vi "RotApp_SaveConfig.vi"(11 "configuration file":path) -> ()   [LabVIEW 2012]
uses:
  RotationProgram/Global/RotationGlobal.vi
  <vilib>/Utility/config.llb/Write Key (Double).vi
  <vilib>/Utility/config.llb/Write Key (String).vi
  <vilib>/Utility/config.llb/Write Key (Path).vi
  <vilib>/Utility/config.llb/NI_LVConfig.lvlib
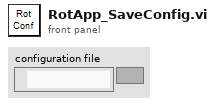
[diagram p1: front panel]
types:
  T1 = typedef "NI_LVConfig.lvlib/Config Data RefNum.ctl" = refnum<k1>
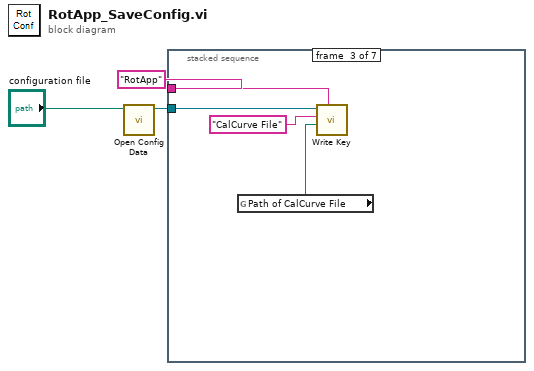
[diagram p0: block diagram]
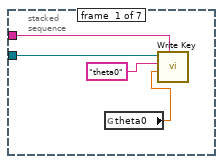
[diagram p2: hidden frame]
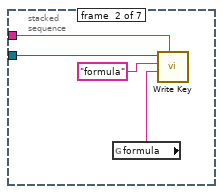
[diagram p3: hidden frame]
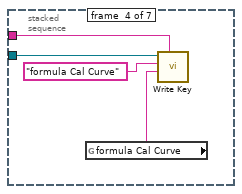
[diagram p4: hidden frame]
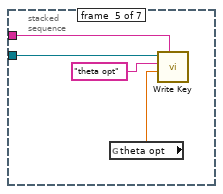
[diagram p5: hidden frame]
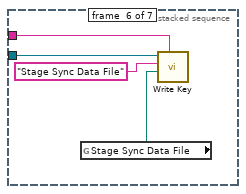
[diagram p6: hidden frame]
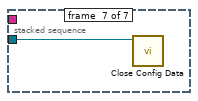
[diagram p7: hidden frame]
diagram:
  n1 = call <vilib>:"Open Config Data.vi"("configuration file path"="configuration file") -> ("refnum"=w2:T1)  [unwired: 8 in, 2 out]
  n2 = stacked-sequence {
    tunnel: w2 -> [w7 w11 w15 w19 w23 w27 w28]
    tunnel: "RotApp" ("section") -> [w6 w10 w14 w18 w22 w26 _]
    frame #0 {
      n3 = global read "RotationGlobal.vi" "theta0"() -> (w4:dbl)
      n4 = call-poly <vilib>:"Write Key.vi"("section"=w6, "value"=w4, "key"="theta0", "refnum"=w7) -> ()  [unwired: 5 in, 3 out]
    }
    frame #1 {
      n5 = global read "RotationGlobal.vi" "formula"() -> (w8:string)
      n6 = call-poly <vilib>:"Write Key.vi"("section"=w10, "value"=w8, "key"="formula", "refnum"=w11) -> ()  [unwired: 5 in, 3 out]
    }
    frame #2 {
      n7 = global read "RotationGlobal.vi" "Path of CalCurve File"() -> (w12:path)
      n8 = call-poly <vilib>:"Write Key.vi"("section"=w14, "value"=w12, "key"="CalCurve File", "refnum"=w15) -> ()  [unwired: 5 in, 3 out]
    }
    frame #3 {
      n9 = global read "RotationGlobal.vi" "formula Cal Curve"() -> (w16:string)
      n10 = call-poly <vilib>:"Write Key.vi"("section"=w18, "value"=w16, "key"="formula Cal Curve", "refnum"=w19) -> ()  [unwired: 5 in, 3 out]
    }
    frame #4 {
      n11 = global read "RotationGlobal.vi" "theta opt"() -> (w20:dbl)
      n12 = call-poly <vilib>:"Write Key.vi"("section"=w22, "value"=w20, "key"="theta opt", "refnum"=w23) -> ()  [unwired: 5 in, 3 out]
    }
    frame #5 {
      n13 = global read "RotationGlobal.vi" "Stage Sync Data File"() -> (w24:path)
      n14 = call-poly <vilib>:"Write Key.vi"("section"=w26, "value"=w24, "key"="Stage Sync Data File", "refnum"=w27) -> ()  [unwired: 5 in, 3 out]
    }
    frame #6 {
      n15 = call <vilib>:"Close Config Data.vi"("refnum"=w28) -> ()  [unwired: 9 in, 2 out]
    }
  }
